vi "Initialize Sequence Call Dictionary.vi"(8 "error in (no error)":errorcluster, 11 "Measurement Interface in":refnum<class "Measurement Interface.lvclass">) -> (0 "error out":errorcluster, 3 "Measurement Interface out":refnum<class "Measurement Interface.lvclass">)   [LabVIEW 2016, in "Measurement Interface.lvlib" / "Measurement Interface.lvclass"]
uses:
  Measurement Interface.lvclass
  Measurement Interface.lvclass/Measurement Interface.ctl
  Engine Reference/Read Engine Reference.vi
  Active Sequence File/Read Active Sequence File.vi
  Sequence Call Step/Write Sequence Call Step Dictionary.vi
  Plugins/Sequence Call Step Dictionary.lvlibp/Sequence Call Step Dictionary.lvclass
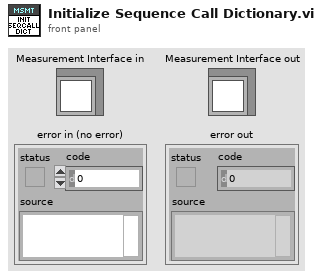
[diagram p1: front panel]
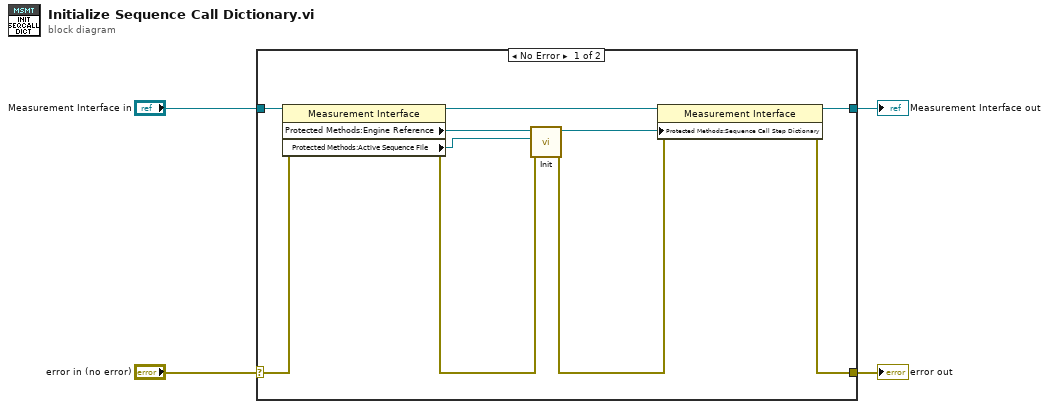
[diagram p0: block diagram]
diagram:
  n1 = case shown="No Error" "error in (no error)" {
    selector: "error in (no error)" -> [w14 w16]
    tunnel: [w8 w16] -> w3
    tunnel: [w6 w15] -> w1
    tunnel: "Measurement Interface in" -> [w13 w15]
    frame No Error {
      n2 = property class="Measurement Interface"(reference=w13, error in=w14) -> (reference out=w7:refnum<class "Measurement Interface.lvclass">, error out=w10:errorcluster, "Protected Methods:Engine Reference"=w12:refnum<k7>, "Protected Methods:Active Sequence File"=w11:refnum<k7>)
      n3 = call "Init.vi"("error in (no error)"=w10, "Active Sequence File"=w11, "Engine In"=w12) -> ("error out"=w9:errorcluster, "Sequence Call Step  Dictionary out"=w5:refnum<class "Sequence Call Step Dictionary.lvclass">)  [unwired: 6 in, 1 out]
      n4 = property class="Measurement Interface"(reference=w7, error in=w9, "Protected Methods:Sequence Call Step Dictionary"=w5) -> (reference out=w6:refnum<class "Measurement Interface.lvclass">, error out=w8:errorcluster)
    }
    frame Error {
    }
  }
  "error out" <- w3
  "Measurement Interface out" <- w1
